vi "Drive To Ball.vi"() -> ()   [LabVIEW 2013]
panel:
  in  "Reinit":bool
  out "Y":dbl
  out "X":dbl
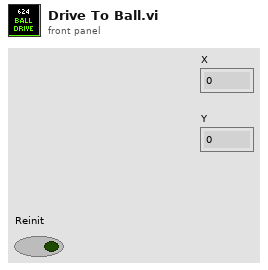
[diagram p1: front panel]
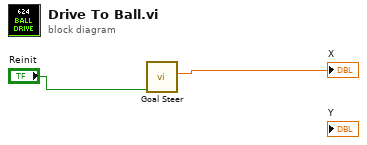
[diagram p0: block diagram]
diagram:
  n1 = call "Goal Steer.vi"("Reinit?"="Reinit") -> ("Steering Out"=→"X":dbl)  [unwired: 10 in]
